vi "bats.parser.ip.vi"() -> ()   [LabVIEW 2020]
uses:
  <vilib>/Platform/TimedLoop/XDataNode/XDataNode.xnode
  <vilib>/Platform/TimedLoop/XDataNode/nitl_modes.ctl
  <vilib>/Platform/TimedLoop/XDataNode/XDNodeRunTimeDep.lvlib
  <vilib>/Platform/TimedLoop/XDataNode/wakeup.ctl
  <vilib>/Platform/TimedLoop/XDataNode/timing_clust.ctl
  <vilib>/rvi/DataTransferAndStorage/Container/XNode/niFpgaContainer.xnode
  <vilib>/rvi/FIFO/Fifo_Resource/nirvififoEmulationRead.vi
panel:
  out "seq no":u32
  out "Remove":bool
  out "Edit":bool
  out "Add":bool
  out "Bytes.Valid":u8
  out "Bytes.echo":u64
  in  "data.valid":bool
  in  "Byte.Enables":bool[](array[boolean])=[FALSE, FALSE, FALSE, FALSE, FALSE, FALSE, FALSE, FALSE]
  in  "Bytes":u8[](array[numeric])=[0, 0, 0, 0, 0, 0, 0, 0] format="%.0x"
  out "Nanoseconds (U64)":u64
  out "Seconds (U64)":u64
  out "Remaining Quantity (U32)":u32
  out "OrderBook Command.Type":T1(ring)
  out "Debug.Valid":bool
  out "Debug.Element":u64
  in  "Ready.For.Debug":bool
  out "OrderBook.Command.Valid":bool
  out "Canceled Quantity (U32)":u32
  out "Executed Quantity (U32)":u32
  out "Price (U64)":u64
  out "Symbol (U64)":u64
  out "Quantity (U32)":u32
  out "Order Id (U64)":u64
  out "Side (U8)":u8
  in  "Ready.for.OrderBook.Command":bool
  out "Ready.for.Udp.Input":bool
  in  "reset":bool
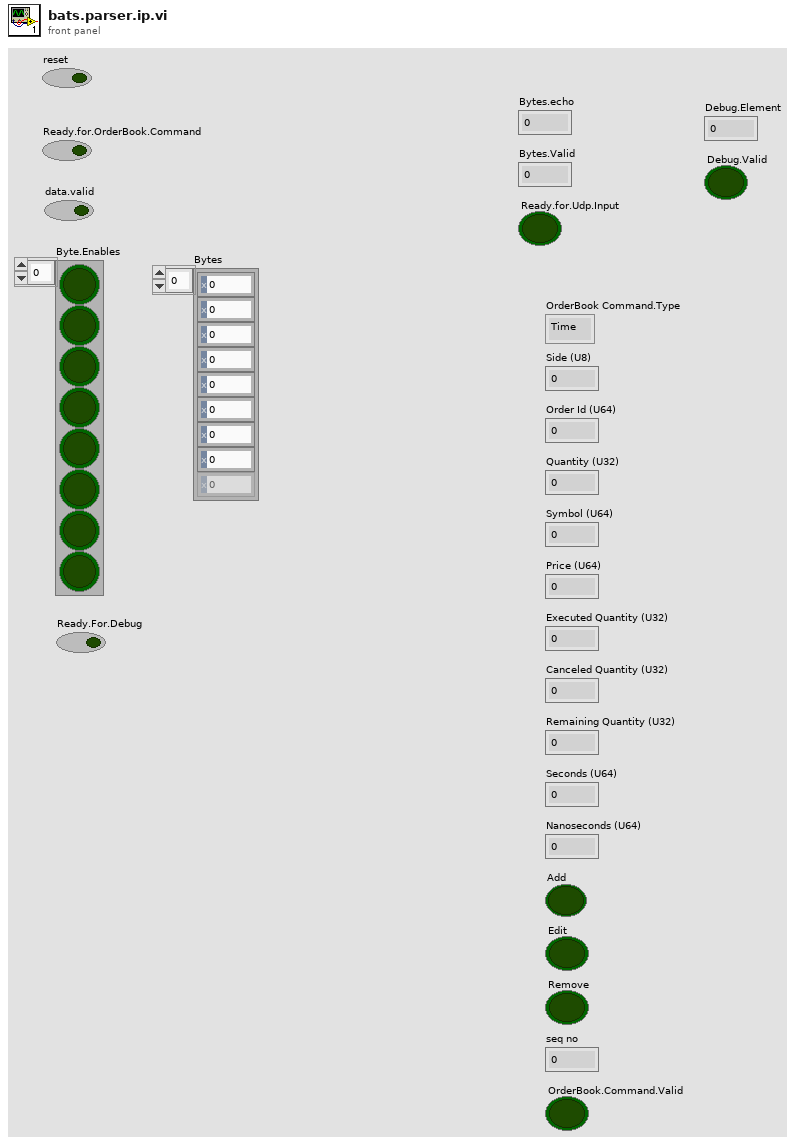
[diagram p1: front panel]
types:
  T1 = enum8{"Time", "AddOrder", "OrderExecuted", "OrderExecutedAtPrice", "ReduceSize", "ModifyOrder", "DeleteOrder", "Get.Everything", "Get.All.Orders", "Get.Top"}
  T2 = typedef "XDNodeRunTimeDep.lvlib/timing_clust.ctl" = cluster{"Expected End [f-1]":u64, "Actual End [f-1]":u64, "Finished Late? [f-1]":bool, "Expected End [i-1]":u64, "Actual End [i-1]":u64, "Finished Late? [i-1]":bool, "Expected Start [i]":u64, "Actual Start [i]":u64, "Expected Start [f]":u64, "Actual Start [f]":u64, "Source Name":string, "Structure Name":string, "Period":i64, "Deadline":i64, "Offset":i64, "Start":i64, "Priority":i32, "Timeout":i32, "Mode":T3, "Wakeup Reason":T4, "Error":errorcluster, "Source Type":string, "Secondary Source Type":string, "Global End Time":u64, "Global Start Time":u64, "Frame Duration":u64, "Iteration Duration":u64, "Assigned CPU":i32, "I/O Scan Engine Mode":u32}
  T3 = typedef "XDNodeRunTimeDep.lvlib/nitl_modes.ctl" = enum32{"No Change", "Process missed periods, maintain original phase", "Discard missed periods, maintain original phase", "Process missed periods, ignore original phase", "Discard missed periods, ignore original phase"}
  T4 = typedef "XDNodeRunTimeDep.lvlib/wakeup.ctl" = enum32{"Normal", "Aborted", "Asynchronous wakeup", "Timing source error", "Timed loop error", "Timeout"}
  T5 = cluster{"type":enum8{"Time", "AddOrder", "OrderExecuted", "OrderExecutedAtPrice", "ReduceSize", "ModifyOrder", "DeleteOrder", "Get.Everything", "Get.All.Orders", "Get.Top"}, "side":u8, "orderId ":u64, "quantity":u32, "symbol":u64, "price":u64, "executed.qty":u32, "canceled.qty":u32, "remaining.qty":u32, "seconds":u64, "nanoseconds":u64, "Add":bool, "Edit":bool, "Remove":bool, "seq no":u32}
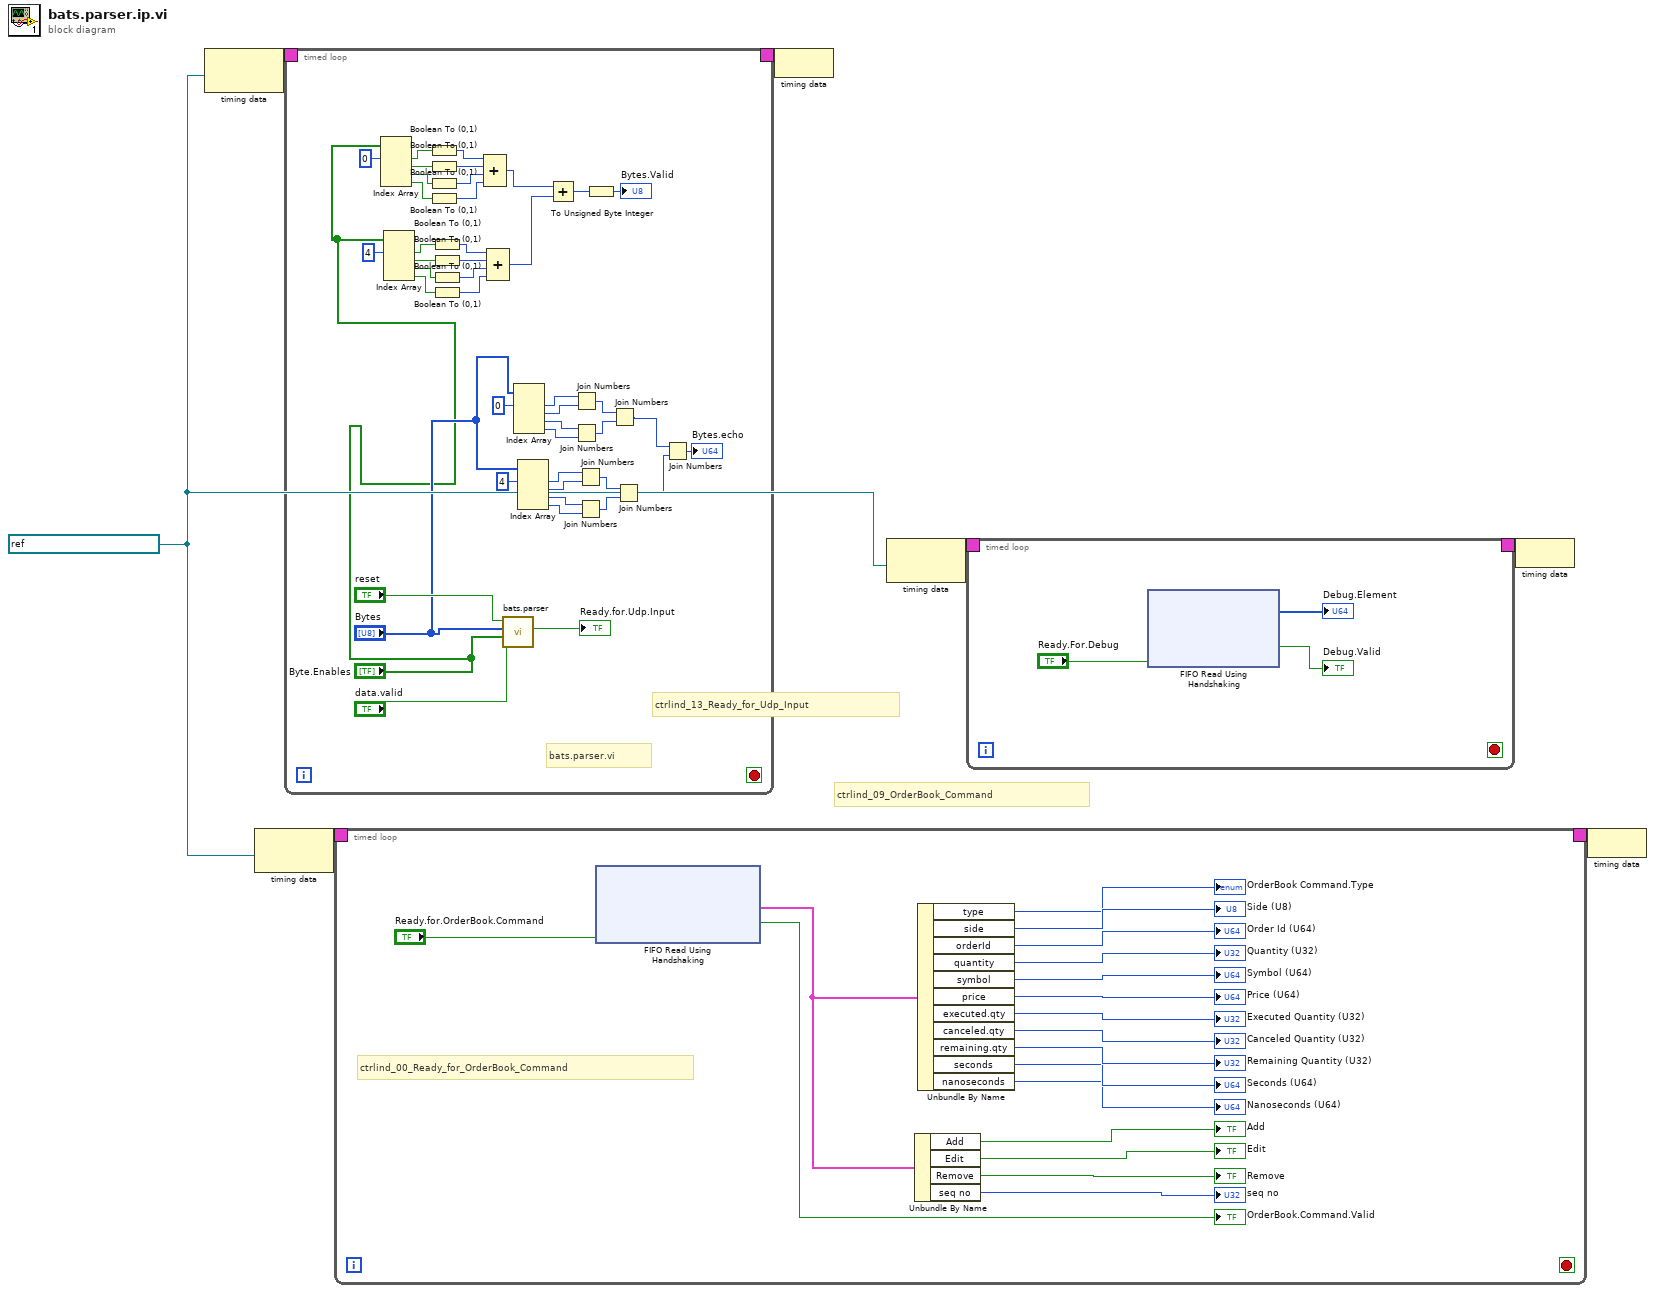
[diagram p0: block diagram]
diagram:
  w1 = refnum<k21> "40 MHz Onboard Clock" ("Source Name")
  # "ctrlind_09_OrderBook_Command"
  # "ctrlind_13_Ready_for_Udp_Input"
  n1 = node-c288(w1) -> (w7:T2)
  n2 = node-c288(w1) -> (w5:T2)
  n3 = timed-loop {
    timing: w7 -> [_]
    timing-out: [_] -> w6
    stop <- _ stop-if-true
    # "bats.parser.vi"
    n4 = Index Array(array="Byte.Enables", index #1=0 ("index")) -> (element #1=w11:bool, element #2=w13:bool, element #3=w15:bool, element #4=w18:bool)  [unwired: 3 in]
    n5 = Index Array(array="Byte.Enables", index #1=4 ("index")) -> (element #1=w21:bool, element #2=w23:bool, element #3=w25:bool, element #4=w28:bool)  [unwired: 3 in]
    n6 = Boolean To (0,1)(Boolean=w11) -> (0, 1=w12:i16)
    n7 = Boolean To (0,1)(Boolean=w13) -> (0, 1=w14:i16)
    n8 = Boolean To (0,1)(Boolean=w15) -> (0, 1=w16:i16)
    n9 = Boolean To (0,1)(Boolean=w18) -> (0, 1=w17:i16)
    n10 = Boolean To (0,1)(Boolean=w21) -> (0, 1=w22:i16)
    n11 = Boolean To (0,1)(Boolean=w23) -> (0, 1=w24:i16)
    n12 = Boolean To (0,1)(Boolean=w25) -> (0, 1=w26:i16)
    n13 = Boolean To (0,1)(Boolean=w28) -> (0, 1=w27:i16)
    n14 = Compound Arithmetic op=ADD(w12, w14, w16, w17) -> (w19:i16)
    n15 = Compound Arithmetic op=ADD(w22, w24, w26, w27) -> (w29:i16)
    n16 = call "bats.parser.vi"(8:"data.valid", "time"="Byte.Enables", "data.stream"="Bytes", "reset"="reset") -> ("Ready.for.Udp.Input"=→"Ready.for.Udp.Input":bool)  [unwired: 7 in]
    n17 = Index Array(array="Bytes", index #1=0 ("index")) -> (element #1=w47:u8, element #2=w46:u8, element #3=w45:u8, element #4=w44:u8)  [unwired: 3 in]
    n18 = Index Array(array="Bytes", index #1=4 ("index")) -> (element #1=w39:u8, element #2=w38:u8, element #3=w37:u8, element #4=w36:u8)  [unwired: 3 in]
    n19 = Add(x=w19, y=w29) -> (x+y=w30:i16)
    n20 = Join Numbers(hi=w47, lo=w46) -> ((hi.lo)=w43:u16)
    n21 = Join Numbers(hi=w45, lo=w44) -> ((hi.lo)=w42:u16)
    n22 = Join Numbers(hi=w39, lo=w38) -> ((hi.lo)=w35:u16)
    n23 = Join Numbers(hi=w37, lo=w36) -> ((hi.lo)=w34:u16)
    n24 = To Unsigned Byte Integer(number=w30) -> (unsigned 8bit integer=→"Bytes.Valid":u8)
    n25 = Join Numbers(hi=w43, lo=w42) -> ((hi.lo)=w41:u32)
    n26 = Join Numbers(hi=w35, lo=w34) -> ((hi.lo)=w33:u32)
    n27 = Join Numbers(hi=w41, lo=w33) -> ((hi.lo)=→"Bytes.echo":u64)
  }
  n28 = timed-loop {
    timing: w5 -> [_]
    timing-out: [_] -> w4
    stop <- _ stop-if-true
    # "ctrlind_00_Ready_for_OrderBook_Command"
    n29 = xnode ("FIFO Read Using Handshaking")("Ready for Output"="Ready.for.OrderBook.Command") -> ("Element"=w58:T5, "Output Valid"=→"OrderBook.Command.Valid":bool)  [unwired: 1 in, 1 out]
    n30 = Unbundle By Name(w58) -> ("Add"=→"Add":bool, "Edit"=→"Edit":bool, "Remove"=→"Remove":bool, "seq no"=→"seq no":u32)
    n31 = Unbundle By Name(w58) -> ("type"=→"OrderBook Command.Type":T1, "side"=→"Side (U8)":u8, "orderId"=→"Order Id (U64)":u64, "quantity"=→"Quantity (U32)":u32, "symbol"=→"Symbol (U64)":u64, "price"=→"Price (U64)":u64, "executed.qty"=→"Executed Quantity (U32)":u32, "canceled.qty"=→"Canceled Quantity (U32)":u32, "remaining.qty"=→"Remaining Quantity (U32)":u32, "seconds"=→"Seconds (U64)":u64, "nanoseconds"=→"Nanoseconds (U64)":u64)
  }
  n32 = node-c288(w6) -> ()
  n33 = node-c288(w1) -> (w3:T2)
  n34 = timed-loop {
    timing: w3 -> [_]
    timing-out: [_] -> w2
    stop <- _ stop-if-true
    n35 = xnode ("FIFO Read Using Handshaking")("Ready for Output"="Ready.For.Debug") -> ("Element"=→"Debug.Element":u64[], "Output Valid"=→"Debug.Valid":bool)  [unwired: 1 in, 1 out]
  }
  n36 = node-c288(w2) -> ()
  n37 = node-c288(w4) -> ()
